vi "Operation Complete Query.vi"(0 "VISA resource name":refnum<visa-resource-name>, 11 "error in (no error)":errorcluster) -> (4 "VISA resource name out":refnum<visa-resource-name>, 6 "Operation Complete":bool caption="Operation Complete?", 15 "error out":errorcluster)   [LabVIEW 2018, in "XP Power PLS600.lvlib"]
doc: "Reads the Operation Complete bit to see if the last operation was completed successully."
uses:
  XP Power PLS600.lvlib
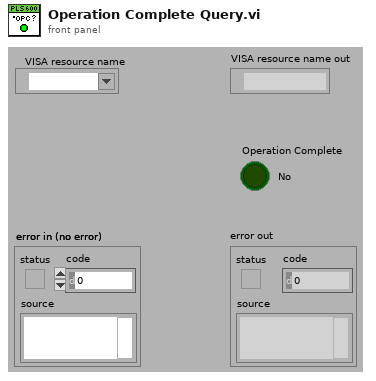
[diagram p1: front panel]
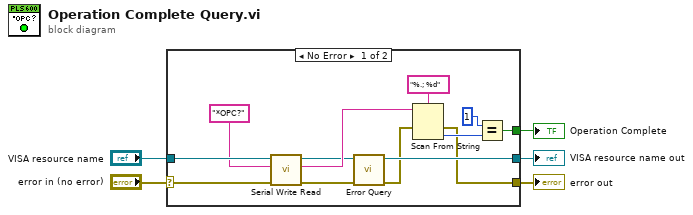
[diagram p0: block diagram]
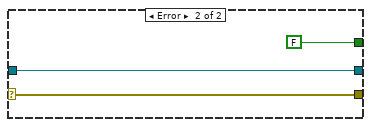
[diagram p2: hidden frame]
diagram:
  n1 = case shown="No Error" "error in (no error)" {
    selector: "error in (no error)" -> [w9 w20]
    tunnel: [w15 FALSE] -> w5
    tunnel: "VISA resource name" -> [w11 w21]
    tunnel: [w12 w20] -> w2
    tunnel: [w14 w21] -> w1
    frame No Error {
      n2 = call "Serial Write Read.vi"("error in (no error)"=w9, "Write Buffer"="*OPC?" ("Command to Send (empty)"), "VISA resource name"=w11) -> ("error out"=w8:errorcluster, "Read Buffer"=w7:string, "VISA resource name out"=w6:refnum<visa-resource-name>)  [unwired: 6 in]
      n3 = call "Error Query.vi"("error in (no error)"=w8, "VISA resource name"=w6) -> ("error out"=w13:errorcluster, "VISA resource name out"=w14:refnum<visa-resource-name>)  [unwired: 6 in, 2 out]
      n4 = Scan From String(format string="%.; %d" ("Format String"), input string=w7, error in=w13) -> (error out=w12:errorcluster, output 1=w17:i32)  [unwired: 2 in, 2 out]
      n5 = Equal?(x=1, y=w17) -> (x = y?=w15:bool)
    }
    frame Error {
    }
  }
  "Operation Complete" <- w5
  "error out" <- w2
  "VISA resource name out" <- w1
